vi "setDescription.vi"(8 "error in (no error)":errorcluster, 10 "description":string="Dark Roast", 11 "DarkRoast in":refnum<class "DarkRoast.lvclass">) -> (0 "error out":errorcluster, 3 "DarkRoast out":refnum<class "DarkRoast.lvclass">)   [LabVIEW 2017, in "DarkRoast.lvclass"]
uses:
  DarkRoast.lvclass
  Beverage Class/Beverage.lvclass
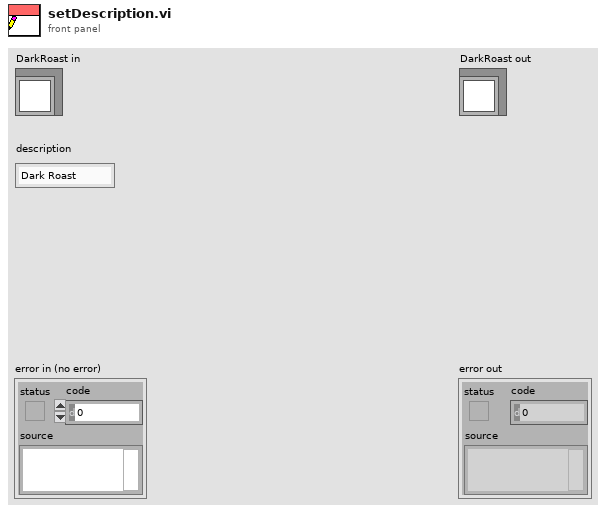
[diagram p1: front panel]
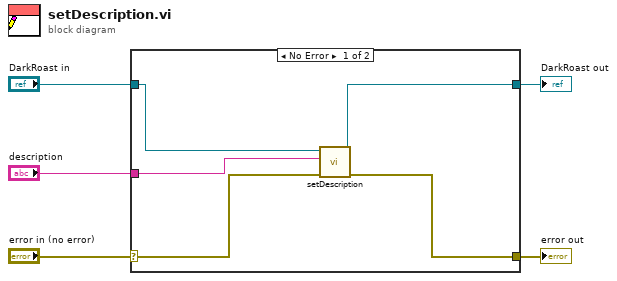
[diagram p0: block diagram]
diagram:
  n1 = case shown="No Error" "error in (no error)" {
    selector: "error in (no error)" -> [w10 w11]
    tunnel: [w9 w11] -> w4
    tunnel: [w7 w12] -> w2
    tunnel: "DarkRoast in" -> [w8 w12]
    tunnel: "description" -> [w6 _]
    frame No Error {
      n2 = call-parent "setDescription.vi"("error in (no error)"=w10, "description"=w6, "Beverage in"=w8) -> ("error out"=w9:errorcluster, "Beverage out"=w7:refnum<class "DarkRoast.lvclass">)  [unwired: 7 in]
    }
    frame Error {
    }
  }
  "error out" <- w4
  "DarkRoast out" <- w2
